vi "Register Endpoint.vi"(8 "error in (no error)":errorcluster, 10 "Stream:Endpoint":refnum<class "Endpoint.lvclass">, 11 "Manager in":refnum<class "Manager.lvclass">) -> (0 "error out":errorcluster, 3 "Manager out":refnum<class "Manager.lvclass">)   [LabVIEW 2020, in "Stream-Simple-Msg.lvlib" / "Manager.lvclass"]
doc: "Registers an underlying Stream Endpoint instance to use for messaging e.g. a TCP Client/Server, WebSocket Client/Server, etc.\n\nOnce an endpoint is registered it no longer needs to be managed by the application; when the manager instance is cleaned up all registered endpoints will be cleaned up as well. Endpoints being used for messaging should not be used separately as it will interfere with the messaging functionality."
uses:
  Manager.lvclass
  <vilib>/IlluminatedG/lv-stream/Endpoint/Endpoint.lvclass
  <vilib>/IlluminatedG/lv-stream/stream/Mode.ctl
  Manager.lvclass/Manager.ctl
  Connection State Callback.vi
  <vilib>/IlluminatedG/lv-stream/Stream.lvlib
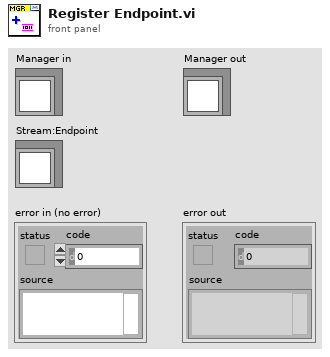
[diagram p1: front panel]
types:
  T1 = typedef "Stream.lvlib/Mode.ctl" = enum16{"Raw", "Buffered", "LineTerm"}
  T2 = typedef "Stream-Simple-Msg.lvlib/Manager.lvclass/Ref Data.ctl" = cluster{"Message Callbacks":map{string, T3[]}, "Endpoints":map{string, refnum<class "Endpoint.lvclass">}, "Stream Endpoints":refnum<class "Endpoint.lvclass">[], "State Callbacks":T4[]}
  T3 = typedef "Stream-Simple-Msg.lvlib/Manager.lvclass/Callback.ctl" = cluster{"VI":refnum<vi>, "Owner":refnum<class>}
  T4 = typedef "Stream-Simple-Msg.lvlib/Manager.lvclass/State Callback.ctl" = cluster{"Owner":refnum<class>, "VI":refnum<vi>}
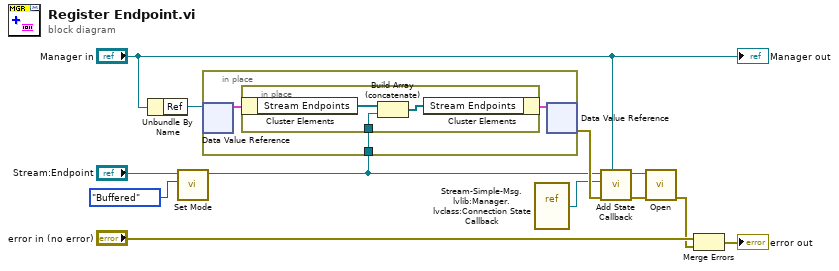
[diagram p0: block diagram]
diagram:
  n1 = Unbundle By Name("Manager in") -> ("Ref"=w8:refnum<data-value>)
  n2 = call <vilib>:"Set Mode.vi"("Mode"=Mode."Buffered", "Endpoint in"="Stream:Endpoint") -> ("Endpoint out"=w1:refnum<class "Endpoint.lvclass">)  [unwired: 8 in, 1 out]
  n3 = in-place {
    in-place-border: w1 -> [w14]
    n4 = in-place-dvr #1(w8) -> (w15:T2)  [unwired: 1 out]
    n5 = in-place {
      in-place-border: w14 -> [w17]
      n6 = in-place-cluster #2(w15) -> ("Stream Endpoints"=w18:refnum<class "Endpoint.lvclass">[])
      n7 = Build Array (concatenate)(w18, w17) -> (w16:refnum<class "Endpoint.lvclass">[])
      n8 = in-place-cluster #2("Stream Endpoints"=w16) -> (w13:T2)
    }
    n9 = in-place-dvr #1(w13) -> (w12:errorcluster)  [unwired: 1 out]
  }
  n10 = vi-ref "Stream-Simple-Msg.lvlib:Manager.lvclass:Connection State Callback.vi"() -> (w10:refnum<vi>)
  n11 = call-dynamic "Add State Callback.vi"("Owner"="Manager in", "error in (no error)"=w12, "Callback"=w10, "Endpoint in"=w1) -> ("error out"=w6:errorcluster, "Endpoint out"=w7:refnum<class "Endpoint.lvclass">)  [unwired: 6 in]
  n12 = call <vilib>:"Open.vi"("error in (no error)"=w6, "Endpoint in"=w7) -> ("error out"=w4:errorcluster)  [unwired: 8 in, 1 out]
  n13 = Merge Errors("error in (no error)", w4) -> (→"error out":errorcluster)
  "Manager out" <- "Manager in"
